vi "Water Pump.vi"(8 "Target Moisture Level":dbl=6.0, 11 "Soil moisture in":u32(slide) scale=0.0..100.0) -> (0 "Soil moisture out":u32, 3 "Checkbox":bool)   [LabVIEW 2021]
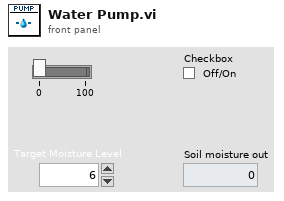
[diagram p1: front panel]
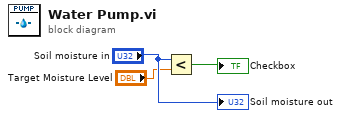
[diagram p0: block diagram]
diagram:
  n1 = Less?(x="Soil moisture in", y="Target Moisture Level") -> (x < y?=→"Checkbox":bool)
  "Soil moisture out" <- "Soil moisture in"
